vi "Rx Inline Start.vi"(8 "error in (no error)":errorcluster, 10 "Dispatcher Interface in":refnum<class "Dispatcher Interface.lvclass">, 11 "Plugin in":refnum<class "Plugin.lvclass">) -> (0 "error out":errorcluster, 2 "Dispatcher Interface out":refnum<class "Dispatcher Interface.lvclass">, 3 "Plugin out":refnum<class "Plugin.lvclass">)   [LabVIEW 2017, in "DSF Core.lvlib" / "Plugin.lvclass"]
uses:
  Plugin.lvclass
  Interfaces/Dispatcher/Dispatcher Interface.lvclass
  C:/Git/DSF/Data Sharing Framework/Source/Core/Engine/Classes/Interfaces/Interface/Interface.lvclass
  Plugin.lvclass/Plugin.ctl
  Interfaces/Dispatcher/Command.ctl
  Transfer Group/Transfer Group.lvclass/Transfer Group.ctl
  Timing/Timing.lvclass/Timing.ctl
  Interfaces/Interface/Interface.lvclass/Interface.ctl
  Interfaces/Dispatcher/Send Dispatcher Command.vi
  Interfaces/Dispatcher/Write.vi
  Interfaces/Dispatcher/Write Dispatcher Command.vi
  Interfaces/Interface/Send Command.vi
  Interfaces/Interface/Write RT FIFO.vi
  Interfaces/Interface/Errors.vi
  Interfaces/Dispatcher/Command Timeout.vi
  VIs/VI Name.vi
  Interfaces/Dispatcher/Class Name.vi
  Transfer Group/Transfer Group.lvclass
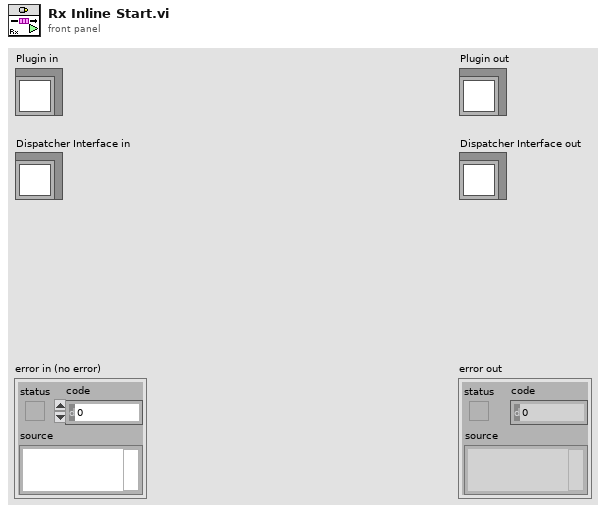
[diagram p1: front panel]
types:
  T1 = typedef "DSF Core.lvlib/Dispatcher Interface.lvclass/Command.ctl" = enum8{"Rx", "Tx", "Set Inline Buffer", "Shutdown"}
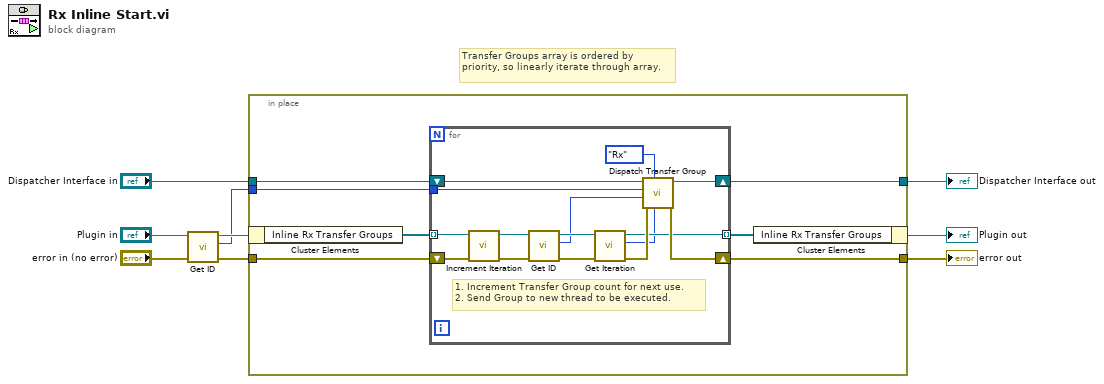
[diagram p0: block diagram]
diagram:
  # "Transfer Groups array is ordered by priority, so linearly iterate through array."
  n1 = call "Get ID.vi"("Plugin in"="Plugin in") -> ("id"=w2:i32, "Plugin out"=w3:refnum<class "Plugin.lvclass">)  [unwired: 9 in]
  n2 = in-place {
    in-place-border: "error in (no error)" -> [w15]
    in-place-border: [w14] -> w8
    in-place-border: "Dispatcher Interface in" -> [w11]
    in-place-border: w2 -> [w10]
    in-place-border: [w9] -> w1
    n3 = in-place-cluster #1(w3) -> ("Inline Rx Transfer Groups"=w13:refnum<class "Transfer Group.lvclass">[])
    n4 = for {
      tunnel: w13 -> [w25] mode=indexing
      shift-right: [w28] -> w14
      shift-left: w15 -> [w26]
      tunnel: [w20] -> w12 mode=indexing
      shift-right: [w23] -> w9
      shift-left: w11 -> [w24]
      tunnel: w10 -> [w22]
      # "1. Increment Transfer Group count for next use.\n2. Send Group to new thread to be executed."
      n5 = call "Increment Iteration.vi"("error in (no error)"=w26, "Transfer Group in"=w25) -> ("error out"=w27:errorcluster, "Transfer Group out"=w16:refnum<class "Transfer Group.lvclass">)  [unwired: 8 in]
      n6 = call "Get ID.vi"("Transfer Group in"=w16) -> ("id"=w19:i32, "Transfer Group out"=w21:refnum<class "Transfer Group.lvclass">)  [unwired: 9 in]
      n7 = call "Get Iteration.vi"("error in (no error)"=w27, "Transfer Group in"=w21) -> ("error out"=w29:errorcluster, "iteration"=w17:u64, "Transfer Group out"=w20:refnum<class "Transfer Group.lvclass">)  [unwired: 7 in]
      n8 = call "Dispatch Transfer Group.vi"("Iteration"=w17, "command"=Command."Rx", "error in (no error)"=w29, "Transfer Group ID"=w19, "Plugin ID"=w22, "Dispatcher Interface in"=w24) -> ("error out"=w28:errorcluster, "Dispatcher Interface out"=w23:refnum<class "Dispatcher Interface.lvclass">)  [unwired: 4 in]
    }
    n9 = in-place-cluster #1("Inline Rx Transfer Groups"=w12) -> (→"Plugin out":refnum<class "Plugin.lvclass">)
  }
  "error out" <- w8
  "Dispatcher Interface out" <- w1
